vi "initialize configuration.vi"(8 "error in":errorcluster, 11 "configuration in":refnum<class "TBM configuration.lvclass">) -> (0 "error out":errorcluster, 2 "instance identifier":string, 3 "configuration out":refnum<class "TBM configuration.lvclass">)   [LabVIEW 2013, in "TBM configuration.lvclass"]
uses:
  TBM configuration.lvclass
  TBM configuration.lvclass/TBM configuration.ctl
  create GUID.vi
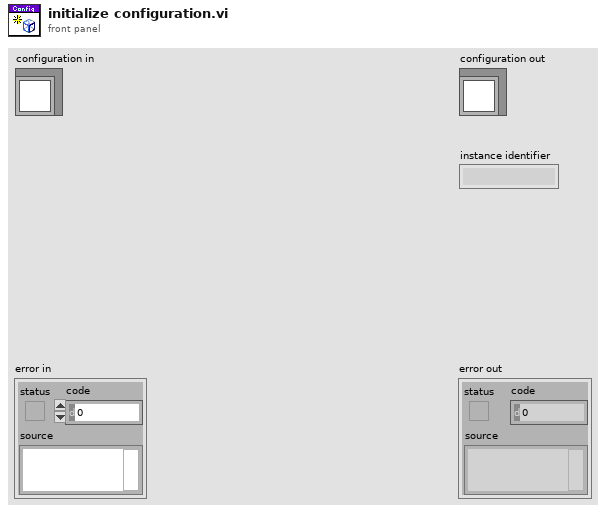
[diagram p1: front panel]
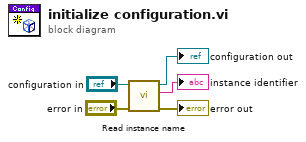
[diagram p0: block diagram]
diagram:
  n1 = call "Read instance name.vi"("error in"="error in", "configuration in"="configuration in") -> ("error out"=→"error out":errorcluster, "instance id"=→"instance identifier":string, "configuration out"=→"configuration out":refnum<class "TBM configuration.lvclass">)  [unwired: 7 in]
